vi "falcon_mps_to_counts.vi"(11 "Velocity (m/s)":dbl) -> (3 "Velocity (Counts/100ms)":dbl)   [LabVIEW 2020]
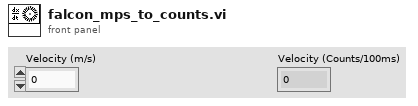
[diagram p1: front panel]
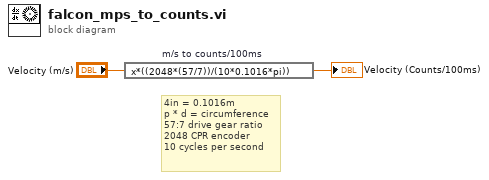
[diagram p0: block diagram]
diagram:
  # "4in = 0.1016m\np * d = circumference\n57:7 drive gear ratio\n2048 CPR encoder\n10 cycles per second"
  n1 = expression code="x*((2048*(57/7))/(10*0.1016*pi))" "m/s to counts/100ms"("Velocity (m/s)") -> (→"Velocity (Counts/100ms)":dbl)
